vi "getGroundAxisAutoOnTarget.vi"(8 "error":errorcluster, 10 "axis":i32, 11 "connection ID":refnum<k5>) -> (0 "error out":errorcluster, 1 "value":bool, 2 "axis_out":i32, 3 "connection ID out":refnum<k5>)   [LabVIEW 2016, in "amc_api.lvlib"]
doc: "Pull axis piezo drive to GND if positioner is in ground target range\n only in AMC300"
uses:
  amc_api.lvlib
panel:
  out "jsonRespIn":string
  out "JSON-response":string="{\"jsonrpc\":\"2.0\",\"method\":\"\",\"params\":[5,1.245,true,\"name\"],\"id\":\"1\"}"
  out "JSON request":string
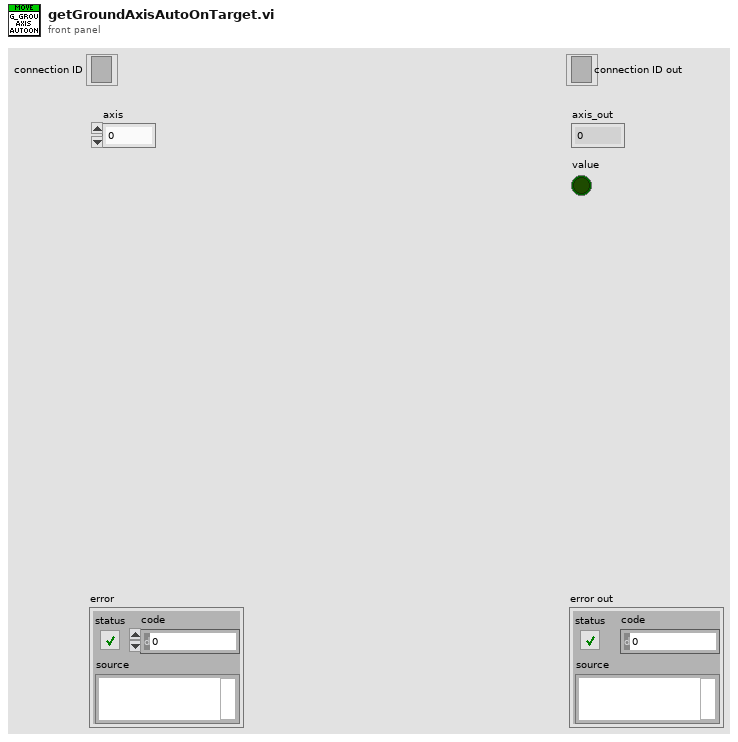
[diagram p1: front panel]
types:
  T1 = cluster{"jsonrpc":string, "method":string, "params":string[], "id":string, "api":i32, "pid":string}
  T2 = enum16{"Standard", "Buffered", "CRLF", "Immediate"}
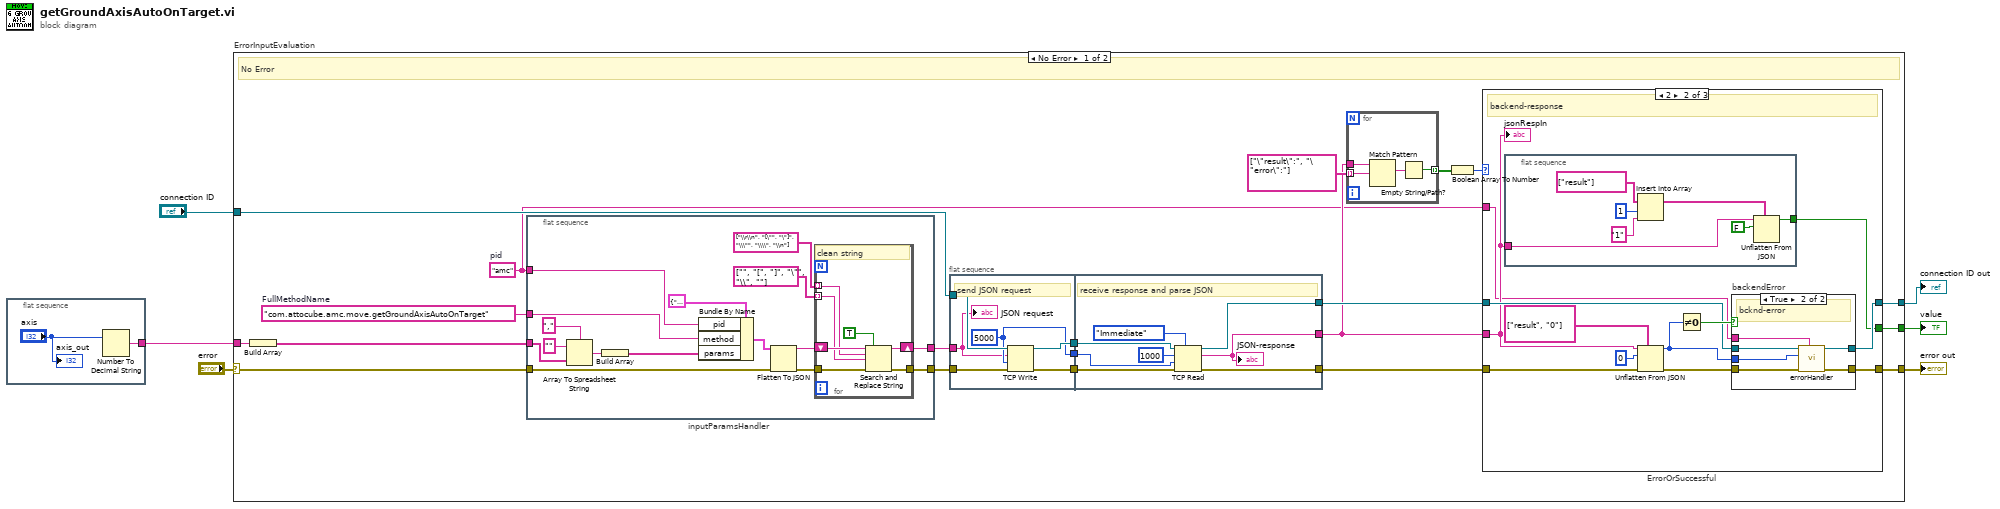
[diagram p0: block diagram]
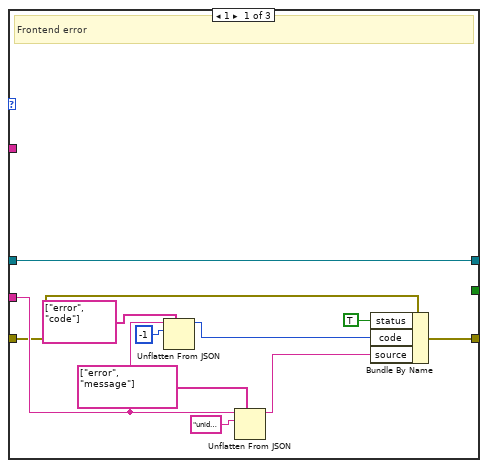
[diagram p2: hidden frame]
diagram:
  n1 = flat-sequence "in_axis" {
    tunnel: [w8] -> w2
    frame #0 {
      n2 = Number To Decimal String(number="axis") -> (decimal integer string=w8:string)  [unwired: 1 in]
      "axis_out" <- "axis"
    }
  }
  n3 = case "ErrorInputEvaluation" shown="No Error" "error" {
    selector: "error" -> [w15 w110]
    tunnel: "connection ID" -> [w25 w111]
    tunnel: [w17 w110] -> w5
    tunnel: [w18 w111] -> w4
    tunnel: w2 -> [w10 _]
    tunnel: [w9 _] -> w1
    frame No Error {
      w11 = "amc"  # pid
      w16 = "com.attocube.amc.move.getGroundAxisAutoOnTarget"  # FullMethodName
      # "No Error"
      n4 = Build Array ("ParametersArrayString")(w10) -> (w14:string[])
      n5 = flat-sequence "inputParamsHandler" {
        tunnel: [w34] -> w13
        tunnel: w14 -> [w40]
        tunnel: w15 -> [w39]
        tunnel: [w36] -> w12
        tunnel: w16 -> [w30]
        tunnel: w11 -> [w29]
        frame #0 {
          n6 = Array To Spreadsheet String(delimiter (Tab)=",", array=w40, 3:"" ("format string")) -> (spreadsheet string=w42:string)
          n7 = Build Array "Build Array"(w42) -> (w31:string[])
          n8 = Bundle By Name(cluster=T1 {"jsonrpc"="2.0", "method"="com.attocube.amc.res.setRESReadOutFreq", "params"=[], "id"="1", "api"=2, "pid"=""}, "pid"=w29, "method"=w30, "params"=w31) -> (w41:T1)
          n9 = Flatten To JSON(anything=w41, error in (no error)=w39) -> (JSON string=w35:string, 11:w37:errorcluster)  [unwired: 1 in]
          n10 = for {
            tunnel: string[] ["\\r\\n", "[\"", "\"]", "\\\"", "\\\\", "\\n"] ("search string") -> [w48] mode=indexing
            tunnel: string[] ["", "[", "]", "\"", "\\", ""] ("replace string (\"\")") -> [w47] mode=indexing
            shift-right: [w50] -> w34
            shift-left: w35 -> [w49]
            tunnel: w37 -> [w46]
            tunnel: [w45] -> w36
            # "clean string"
            n11 = Search and Replace String(replace all?=TRUE ("replace all? (F)"), input string=w49, search string=w48, replace string=w47, error in=w46) -> (result string=w50:string, error out=w45:errorcluster)  [unwired: 3 in, 2 out]
          }
        }
      }
      n12 = flat-sequence {
        tunnel: w25 -> [w101]
        tunnel: [w99] -> w28
        tunnel: [w100] -> w27
        tunnel: w12 -> [w96]
        tunnel: [w98] -> w26
        tunnel: w13 -> [w97]
        tunnel: [w105] -> w21
        tunnel: w28 -> [w107]
        tunnel: w27 -> [w106]
        tunnel: [w103] -> w20
        tunnel: w26 -> [w104]
        tunnel: [w102] -> w19
        frame #0 {
          w98 = 5000 ("timeout ms (25000)")
          # "send JSON request"
          n13 = TCP Write(connection ID=w101, data in=w97, error in (no error)=w96, 9:w98) -> (connection ID out=w99:refnum<k5>, error out=w100:errorcluster)  [unwired: 1 out]
          "JSON request" <- w97
        }
        frame #1 {
          # "receive response and parse JSON"
          n14 = TCP Read(connection ID=w107, bytes to read=1000, error in (no error)=w106, 7:T2."Immediate" ("mode (standard)"), 9:w104) -> (connection ID out=w105:refnum<k5>, data out=w102:string, error out=w103:errorcluster)
          "JSON-response" <- w102
        }
      }
      n15 = for {
        tunnel: string[] ["\"result\":", "\"error\":"] ("path") -> [w54] mode=indexing
        tunnel: [w52] -> w23 mode=indexing
        tunnel: w19 -> [w55]
        n16 = Match Pattern(string=w55, regular expression=w54) -> (match substring=w53:string)  [unwired: 1 in, 3 out]
        n17 = Empty String/Path?(string/path=w53) -> (empty?=w52:bool)
      }
      n18 = Boolean Array To Number(Boolean array=w23) -> (number=w22:u32)
      n19 = case "ErrorOrSuccessful" shown="2" w22 {
        tunnel: w19 -> [w58 w69 _]
        tunnel: w21 -> [w56 w72 w95]
        tunnel: [w56 w71 w95] -> w18
        tunnel: [w59 w70 w94] -> w17
        tunnel: w20 -> [w57 w73 w94]
        tunnel: w11 -> [_ w68 _]
        tunnel: [_ w67 _] -> w9
        frame 1 {
          # "Frontend error"
          n20 = Unflatten From JSON(path=string[] ["error", "code"], JSON string=w58, type and defaults=-1) -> (value=w65:i32)  [unwired: 4 in, 1 out]
          n21 = Unflatten From JSON(path=string[] ["error", "message"], JSON string=w58, type and defaults="unidentified error") -> (value=w66:string)  [unwired: 4 in, 1 out]
          n22 = Bundle By Name(cluster=w57, "status"=TRUE, "code"=w65, "source"=w66) -> (w59:errorcluster)
        }
        frame 2 {
          # "backend-response"
          n23 = flat-sequence "out_bool" {
            tunnel: w69 -> [w84]
            tunnel: [w79] -> w67
            frame #0 {
              n24 = Insert Into Array "Insert Into Array"(array=string[] ["result"] ("path"), index=1, new element="1" ("idx")) -> (w81:string[])
              n25 = Unflatten From JSON(path=w81, JSON string=w84, type and defaults=FALSE) -> (value=w79:bool)  [unwired: 4 in, 1 out]
            }
          }
          n26 = Unflatten From JSON(path=string[] ["result", "0"], JSON string=w69, type and defaults=0, error in (no error)=w73) -> (value=w78:i32, error out=w76:errorcluster)  [unwired: 3 in]
          n27 = Not Equal To 0?(x=w78) -> (x != 0?=w77:bool)
          n28 = case "backendError" shown="True" w77 {
            tunnel: w78 -> [_ w93]
            tunnel: w76 -> [w87 w92]
            tunnel: [w86 w91] -> w71
            tunnel: [w87 w90] -> w70
            tunnel: w72 -> [w86 w89]
            tunnel: w68 -> [_ w88]
            frame False {
              # "successful"
            }
            frame True {
              # "bcknd-error"
              n29 = call "errorHandler.vi"("pid"=w88, "error in"=w92, "errNbr"=w93, "connection ID"=w89) -> ("error out 2"=w90:errorcluster, "connection ID out"=w91:refnum<k5>)  [unwired: 6 in]
            }
          }
          "jsonRespIn" <- w69
        }
        frame Default {
          # "NoResponse"
        }
      }
    }
    frame Error {
      # "Error"
    }
  }
  "error out" <- w5
  "connection ID out" <- w4
  "value" <- w1
